vi "testAbsangle.vi"() -> ()   [LabVIEW 2012]
doc: "Tests the abs angle function. Successful."
uses:
  Data/TypeDefs/UTM Location.ctl
panel:
  out "Angle between points":dbl
  in  "Point 1":T1 {"North" format="%#_10f"; "East" format="%#_8f"}
  in  "Point 2":T1 {"North" format="%#_10f"; "East" format="%#_8f"}
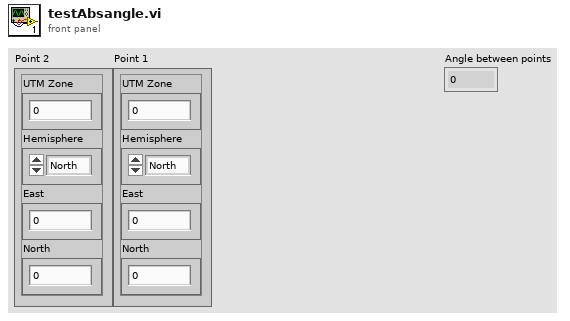
[diagram p1: front panel]
types:
  T1 = typedef "UTM Location.ctl" = cluster{"UTM Zone":dbl, "Hemisphere":enum16{"North", "South"}, "East":dbl, "North":dbl}
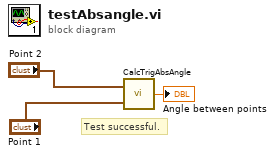
[diagram p0: block diagram]
diagram:
  # "Test successful."
  n1 = call "CalcTrigAbsAngle.vi"("Point 1"="Point 1", "Point 2"="Point 2") -> ("Angle between points"=→"Angle between points":dbl)
